vi "setup_name_dialog.vi"(8 "error in (no error)":errorcluster, 10 "Setup name":string) -> (0 "error out":errorcluster, 2 "setup name":string)   [LabVIEW 2010]
panel:
  in  "okButton":bool
  # "Please enter the setup name:"
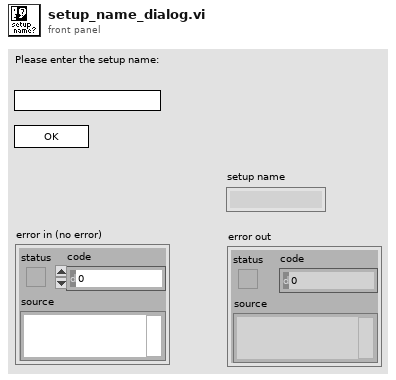
[diagram p1: front panel]
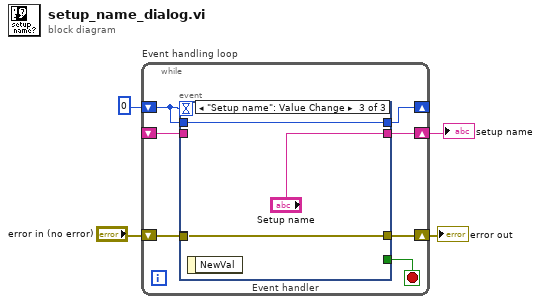
[diagram p0: block diagram]
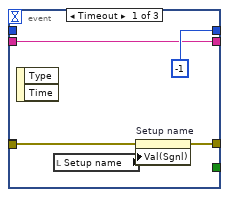
[diagram p2: hidden frame]
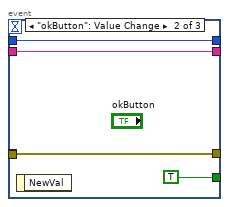
[diagram p3: hidden frame]
diagram:
  n1 = while "Event handling loop" {
    shift-right: [w10] -> w3
    shift-left: "error in (no error)" -> [w11]
    shift-right: [w8] -> w2
    shift-left: _ -> [w9]
    shift-right: [w5] -> _
    shift-left: 0 -> [w6]
    stop <- w7 stop-if-true
    n2 = event "Event handler" shown="[2] \"Setup name\": Value Change" {
      selector: _ -> [_ _ _]
      dyn-events: _ -> [_ _ _]
      timeout: w6 -> [_ _ _]
      tunnel: w11 -> [w15 w20 w23]
      tunnel: w11 -> [_ _ _]
      tunnel: [w14 w20 w23] -> w10
      tunnel: w9 -> [w12 w19 _]
      tunnel: [w12 w19 "Setup name"] -> w8
      tunnel: [_ TRUE _] -> w7
      tunnel: [-1 w17 w21] -> w5
      tunnel: w6 -> [_ w17 w21]
      event Timeout {
        n3 = event-data() -> ()  [unwired: 1 in, 2 out]
        n4 = local read "Setup name"() -> (w13:string)
        n5 = property on="Setup name" class="Str"(error in=w15, "Val(Sgnl)"=w13) -> (error out=w14:errorcluster)  [unwired: 1 in, 1 out]
      }
      event "okButton": Value Change {
        n6 = event-data() -> ()  [unwired: 1 in, 1 out]
      }
      event "Setup name": Value Change {
        n7 = event-data() -> ()  [unwired: 1 in, 1 out]
      }
    }
  }
  "error out" <- w3
  "setup name" <- w2
